vi "playsound.vi"(11 "Play?":cluster{"Warning":bool, "Alarm":bool}={"Warning"=FALSE, "Alarm"=TRUE}) -> ()   [LabVIEW 2019]
panel:
  in  "Stop Button":bool
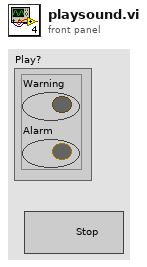
[diagram p1: front panel]
types:
  T1 = typedef "Sound Output Task ID.ctl" = u32
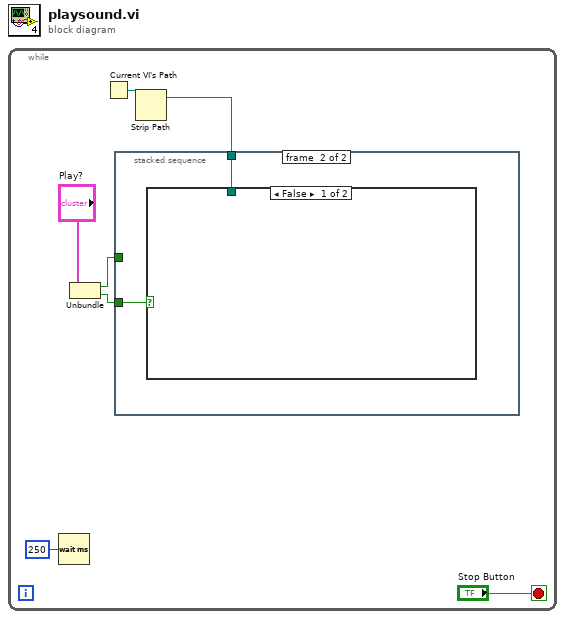
[diagram p0: block diagram]
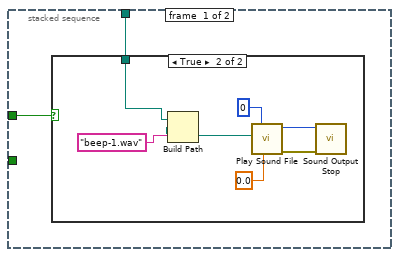
[diagram p2: hidden frame]
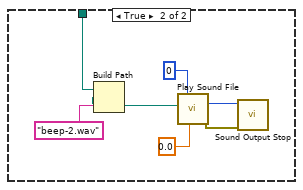
[diagram p4: hidden frame]
diagram:
  n1 = while {
    stop <- "Stop Button" stop-if-true
    n2 = Wait (ms)(milliseconds to wait=u32 250) -> ()  [unwired: 1 out]
    n3 = Unbundle("Play?") -> ("Warning"=w4:bool, "Alarm"=w3:bool)
    n4 = Current VI's Path() -> (path=w7:path)
    n5 = Strip Path(path=w7) -> (stripped path=w6:path)  [unwired: 1 out]
    n6 = stacked-sequence {
      tunnel: w6 -> [w9 w18]
      tunnel: w4 -> [w8 _]
      tunnel: w3 -> [_ w17]
      frame #0 {
        n7 = case shown="True" w8 {
          tunnel: w9 -> [_ w10]
          frame False {
          }
          frame True {
            n8 = Build Path(base path=w10, name or relative path="beep-1.wav") -> (appended path=w15:path)
            n9 = call <vilib>:"Play Sound File.vi"("timeout (sec)"=0.0, "path"=w15, "device ID"=u32 0) -> ("error out"=w11:errorcluster, "task ID"=w12:T1)  [unwired: 7 in]
            n10 = call <vilib>:"Sound Output Stop.vi"("error in (no error)"=w11, "task ID"=w12) -> ()  [unwired: 8 in, 2 out]
          }
        }
      }
      frame #1 {
        n11 = case shown="False" w17 {
          tunnel: w18 -> [_ w21]
          frame False {
          }
          frame True {
            n12 = Build Path(base path=w21, name or relative path="beep-2.wav") -> (appended path=w24:path)
            n13 = call <vilib>:"Play Sound File.vi"("timeout (sec)"=0.0, "path"=w24, "device ID"=u32 0) -> ("error out"=w19:errorcluster, "task ID"=w20:T1)  [unwired: 7 in]
            n14 = call <vilib>:"Sound Output Stop.vi"("error in (no error)"=w19, "task ID"=w20) -> ()  [unwired: 8 in, 2 out]
          }
        }
      }
    }
  }
